vi "ATF Storage-DI Start.vi"(8 "error in":errorcluster, 9 "DI config":T1(array[cluster]), 11 "Refnum in":refnum<k21>) -> (0 "error out":errorcluster, 3 "Refnum out":refnum<k21>)   [LabVIEW 2022 SP3]
doc: "This VI is for start for Analog Output"
uses:
  <vilib>/DAQmx/configure/timing.llb/DAQmx Timing (Sample Clock).vi
  <vilib>/DAQmx/configure/trigger.llb/DAQmx Start Trigger (Time).vi
panel:
  out "Start time 2":timestamp
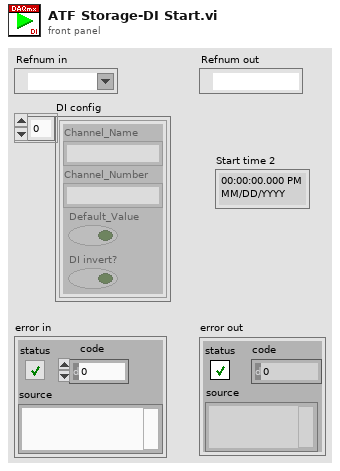
[diagram p1: front panel]
types:
  T1 = cluster{"Channel_Name":string, "Channel_Number":string, "Default_Value":bool, "DI invert?":bool}[]
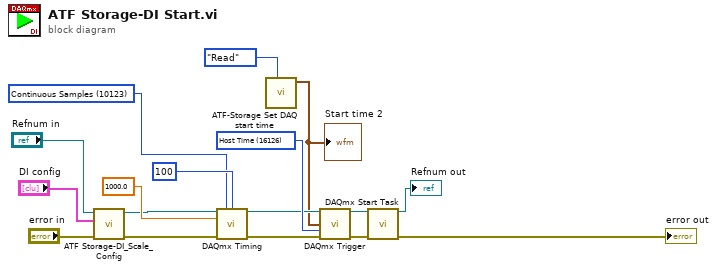
[diagram p0: block diagram]
diagram:
  w8 = 10123 items=["Finite Samples"=10178, "Continuous Samples"=10123, "Hardware Timed Single Point"=12522] ("sample mode")
  w13 = 16126 items=["Host Time"=16126, "I/O Device Time"=16127] ("timescale")
  n1 = call "ATF Storage-DI_Scale_Config.vi"("error in (no error)"="error in", "DI config"="DI config", "Refnum in"="Refnum in") -> ("error out"=w6:errorcluster, "Refnum out"=w7:refnum<k21>)  [unwired: 7 in]
  n2 = call-poly <vilib>:"DAQmx Timing.vi"("task/channels in"=w7, "sample mode"=w8, "samples per channel"=100, "rate"=1000.0, "error in"=w6) -> ("task out"=w12:refnum<k21>, "error out"=w11:errorcluster)  [unwired: 9 in]
  n3 = call "ATF-Storage Set DAQ start time.vi"("Enum"=enum16{"Read", "Write"}."Read") -> ("Start time 2"=w2:timestamp)  [unwired: 10 in]
  "Start time 2" <- w2
  n4 = call-poly <vilib>:"DAQmx Trigger.vi"("task/channels in"=w12, "when"=w2, "timescale"=w13, "error in"=w11) -> ("task out"=w4:refnum<k21>, "error out"=w5:errorcluster)  [unwired: 10 in]
  n5 = call <vilib>:"DAQmx Start Task.vi"("task/channels in"=w4, "error in"=w5) -> ("task out"=→"Refnum out":refnum<k21>, "error out"=→"error out":errorcluster)  [unwired: 12 in]
